vi "Configure Band Marker.vi"(0 "VISA resource name":refnum<visa-resource-name>, 1 "Enable Coupling (Disable)":bool, 2 "Sweep Type (1: Span/Center)":enum16{"Start/Stop", "Span/Center"}(ring)=enum."Span/Center", 3 "Start/Center (0)":dbl format="%^#_9g", 5 "Measurement Type (6: Phase Noise)":u16(ring)=6 items=["AM Noise"=1, "Baseband Noise"=2, "Freq/Power"=3, "Spectrum"=4, "Transient"=5, "Phase Noise"=6, "User"=7], 7 "Select Trace (1: 1)":u16(ring)=1 items=["1"=1, "2"=2, "3"=3, "4"=4, "5"=5, "6"=6, "7"=7, "8"=8], 9 "Select Band Marker (0: Band Marker X)":enum16{"Band Marker X", "Band Marker Y"}(ring), 11 "error in (no error)":errorcluster, 12 "Enable Band Marker (Enable)":bool=TRUE, 13 "Stop/Span (2E12)":dbl=2000000000000.0 format="%^#_9g") -> (4 "VISA resource name out":refnum<visa-resource-name>, 15 "error out":errorcluster)   [LabVIEW 2011, in "Agilent E5052X.lvlib"]
doc: "Configures band markers to be used in measurements. Band markers can be used to limit the range in which analysis or limit test measurements are taken."
uses:
  Agilent E5052X.lvlib
panel:
  # "Band Marker Settings"
  # "Band Marker Sweep Settings"
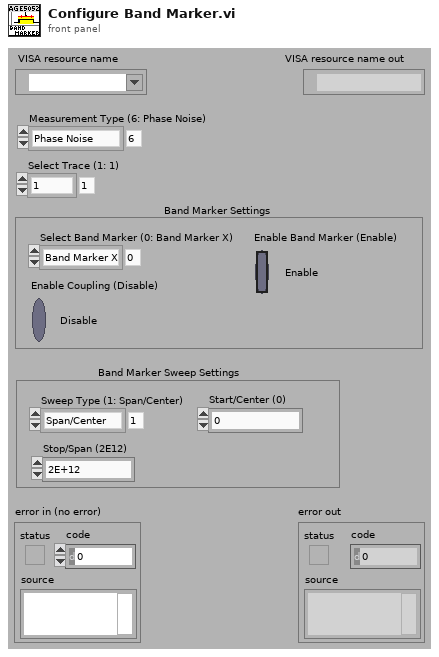
[diagram p1: front panel]
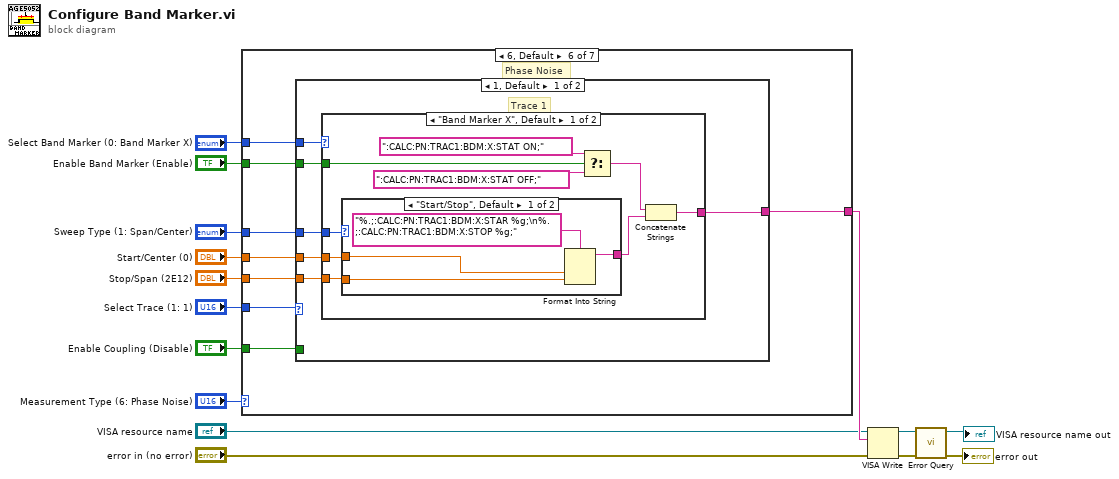
[diagram p0: block diagram]
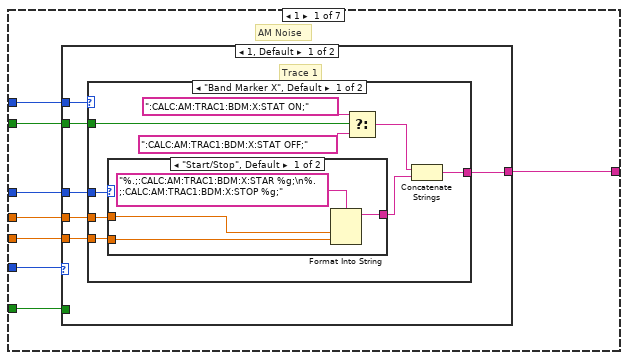
[diagram p2: hidden frame]
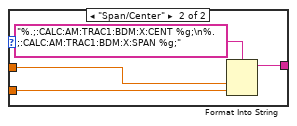
[diagram p3: hidden frame]
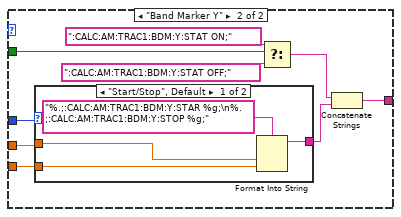
[diagram p4: hidden frame]
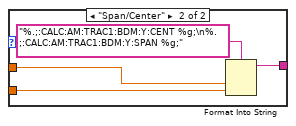
[diagram p5: hidden frame]
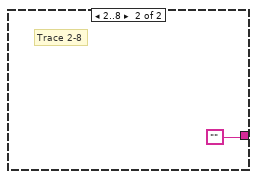
[diagram p6: hidden frame]
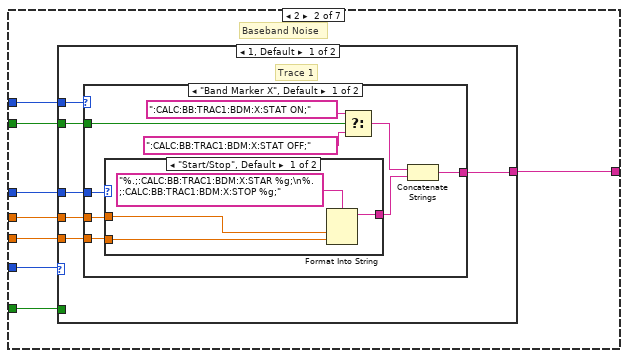
[diagram p7: hidden frame]
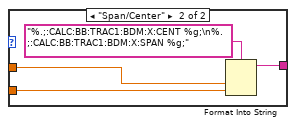
[diagram p8: hidden frame]
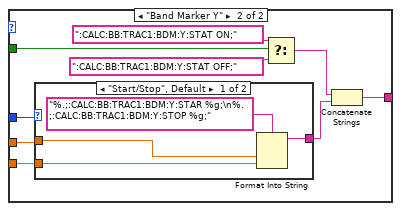
[diagram p9: hidden frame]
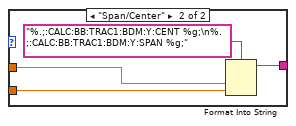
[diagram p10: hidden frame]
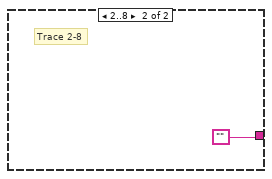
[diagram p11: hidden frame]
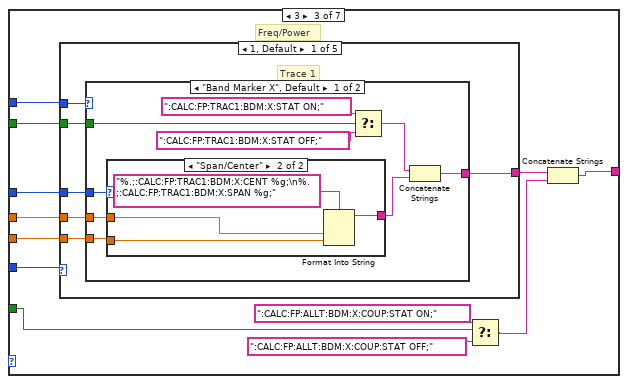
[diagram p12: hidden frame]
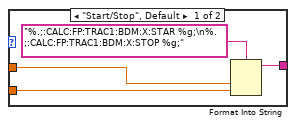
[diagram p13: hidden frame]
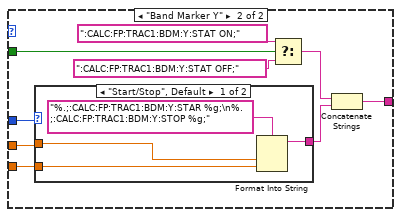
[diagram p14: hidden frame]
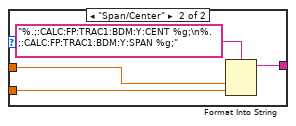
[diagram p15: hidden frame]
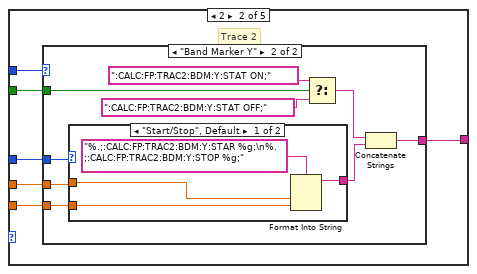
[diagram p16: hidden frame]
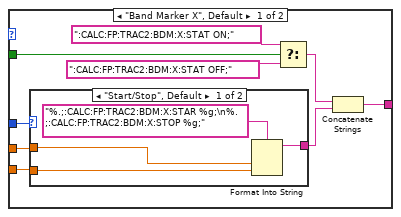
[diagram p17: hidden frame]
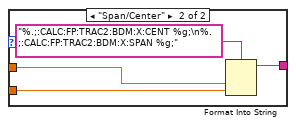
[diagram p18: hidden frame]
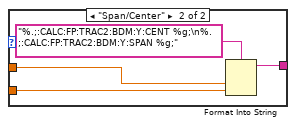
[diagram p19: hidden frame]
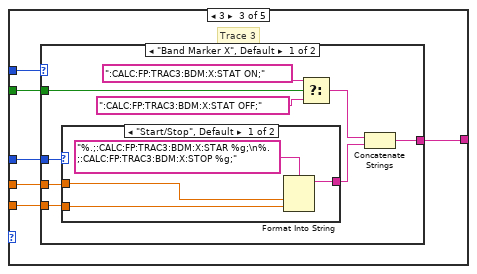
[diagram p20: hidden frame]
diagram:
  n1 = case shown="6, Default" "Measurement Type (6: Phase Noise)" {
    tunnel: "Select Band Marker (0: Band Marker X)" -> [w23 w72 w125 w289 w347 w516 w568]
    tunnel: "Select Trace (1: 1)" -> [w22 w67 w121 w293 w343 w512 w565]
    tunnel: "Enable Coupling (Disable)" -> [w21 w68 w115 w294 w337 w511 w559]
    tunnel: "Start/Center (0)" -> [w20 w70 w123 w291 w345 w514 w566]
    tunnel: "Stop/Span (2E12)" -> [w19 w69 w122 w292 w344 w513 w564]
    tunnel: "Sweep Type (1: Span/Center)" -> [w18 w71 w124 w290 w346 w515 w567]
    tunnel: [w17 w66 w120 w288 w342 w510 w569] -> w7
    tunnel: "Enable Band Marker (Enable)" -> [w16 w65 w118 w287 w340 w509 w562]
    frame 1 {
      # "AM Noise"
      n2 = case shown="1, Default" w22 {
        tunnel: w23 -> [w29 _]
        tunnel: w21 -> [_ _]
        tunnel: w20 -> [w27 _]
        tunnel: w19 -> [w26 _]
        tunnel: w18 -> [w28 _]
        tunnel: [w25 ""] -> w17
        tunnel: w16 -> [w24 _]
        frame 1, Default {
          # "Trace 1"
          n3 = case shown="\"Band Marker X\", Default" w29 {
            tunnel: w28 -> [w38 w55]
            tunnel: w27 -> [w37 w54]
            tunnel: w26 -> [w36 w53]
            tunnel: [w35 w51] -> w25
            tunnel: w24 -> [w32 w48]
            frame "Band Marker X", Default {
              n4 = case shown="\"Start/Stop\", Default" w38 {
                tunnel: w37 -> [w41 w45]
                tunnel: w36 -> [w42 w44]
                tunnel: [w39 w43] -> w34
                frame "Start/Stop", Default {
                  n5 = Format Into String(format string="%.;:CALC:AM:TRAC1:BDM:X:STAR %g;\n%.;:CALC:AM:TRAC1:BDM:X:STOP %g;", w41, w42) -> (resulting string=w39:string)  [unwired: 2 in, 1 out]
                }
                frame "Span/Center" {
                  n6 = Format Into String(format string="%.;:CALC:AM:TRAC1:BDM:X:CENT %g;\n%.;:CALC:AM:TRAC1:BDM:X:SPAN %g;", w45, w44) -> (resulting string=w43:string)  [unwired: 2 in, 1 out]
                }
              }
              n7 = Select(t=":CALC:AM:TRAC1:BDM:X:STAT ON;", s=w32, f=":CALC:AM:TRAC1:BDM:X:STAT OFF;") -> (s? t:f=w31:string)
              n8 = Concatenate Strings(w31, w34) -> (w35:string)
            }
            frame "Band Marker Y" {
              n9 = case shown="\"Start/Stop\", Default" w55 {
                tunnel: w54 -> [w58 w62]
                tunnel: w53 -> [w59 w61]
                tunnel: [w56 w60] -> w52
                frame "Start/Stop", Default {
                  n10 = Format Into String(format string="%.;:CALC:AM:TRAC1:BDM:Y:STAR %g;\n%.;:CALC:AM:TRAC1:BDM:Y:STOP %g;", w58, w59) -> (resulting string=w56:string)  [unwired: 2 in, 1 out]
                }
                frame "Span/Center" {
                  n11 = Format Into String(format string="%.;:CALC:AM:TRAC1:BDM:Y:CENT %g;\n%.;:CALC:AM:TRAC1:BDM:Y:SPAN %g;", w62, w61) -> (resulting string=w60:string)  [unwired: 2 in, 1 out]
                }
              }
              n12 = Select(t=":CALC:AM:TRAC1:BDM:Y:STAT ON;", s=w48, f=":CALC:AM:TRAC1:BDM:Y:STAT OFF;") -> (s? t:f=w47:string)
              n13 = Concatenate Strings(w47, w52) -> (w51:string)
            }
          }
        }
        frame 2..8 {
          # "Trace 2-8"
        }
      }
    }
    frame 2 {
      # "Baseband Noise"
      n14 = case shown="1, Default" w67 {
        tunnel: w72 -> [w78 _]
        tunnel: w68 -> [_ _]
        tunnel: w70 -> [w76 _]
        tunnel: w69 -> [w75 _]
        tunnel: w71 -> [w77 _]
        tunnel: [w74 ""] -> w66
        tunnel: w65 -> [w73 _]
        frame 1, Default {
          # "Trace 1"
          n15 = case shown="\"Band Marker X\", Default" w78 {
            tunnel: w77 -> [w87 w104]
            tunnel: w76 -> [w86 w103]
            tunnel: w75 -> [w85 w102]
            tunnel: [w84 w100] -> w74
            tunnel: w73 -> [w80 w97]
            frame "Band Marker X", Default {
              n16 = case shown="\"Start/Stop\", Default" w87 {
                tunnel: w86 -> [w90 w94]
                tunnel: w85 -> [w91 w93]
                tunnel: [w88 w92] -> w83
                frame "Start/Stop", Default {
                  n17 = Format Into String(format string="%.;:CALC:BB:TRAC1:BDM:X:STAR %g;\n%.;:CALC:BB:TRAC1:BDM:X:STOP %g;", w90, w91) -> (resulting string=w88:string)  [unwired: 2 in, 1 out]
                }
                frame "Span/Center" {
                  n18 = Format Into String(format string="%.;:CALC:BB:TRAC1:BDM:X:CENT %g;\n%.;:CALC:BB:TRAC1:BDM:X:SPAN %g;", w94, w93) -> (resulting string=w92:string)  [unwired: 2 in, 1 out]
                }
              }
              n19 = Select(t=":CALC:BB:TRAC1:BDM:X:STAT ON;", s=w80, f=":CALC:BB:TRAC1:BDM:X:STAT OFF;") -> (s? t:f=w79:string)
              n20 = Concatenate Strings(w79, w83) -> (w84:string)
            }
            frame "Band Marker Y" {
              n21 = case shown="\"Start/Stop\", Default" w104 {
                tunnel: w103 -> [w107 w111]
                tunnel: w102 -> [w108 w110]
                tunnel: [w105 w109] -> w101
                frame "Start/Stop", Default {
                  n22 = Format Into String(format string="%.;:CALC:BB:TRAC1:BDM:Y:STAR %g;\n%.;:CALC:BB:TRAC1:BDM:Y:STOP %g;", w107, w108) -> (resulting string=w105:string)  [unwired: 2 in, 1 out]
                }
                frame "Span/Center" {
                  n23 = Format Into String(format string="%.;:CALC:BB:TRAC1:BDM:Y:CENT %g;\n%.;:CALC:BB:TRAC1:BDM:Y:SPAN %g;", w111, w110) -> (resulting string=w109:string)  [unwired: 2 in, 1 out]
                }
              }
              n24 = Select(t=":CALC:BB:TRAC1:BDM:Y:STAT ON;", s=w97, f=":CALC:BB:TRAC1:BDM:Y:STAT OFF;") -> (s? t:f=w96:string)
              n25 = Concatenate Strings(w96, w101) -> (w100:string)
            }
          }
        }
        frame 2..8 {
          # "Trace 2-8"
        }
      }
    }
    frame 3 {
      # "Freq/Power"
      n26 = case shown="1, Default" w121 {
        tunnel: w125 -> [w131 w171 w210 w251 _]
        tunnel: w123 -> [w129 w169 w208 w249 _]
        tunnel: w122 -> [w128 w168 w207 w248 _]
        tunnel: w124 -> [w130 w170 w209 w250 _]
        tunnel: [w127 w167 w211 w247 ""] -> w119
        tunnel: w118 -> [w126 w166 w206 w246 _]
        frame 1, Default {
          # "Trace 1"
          n27 = case shown="\"Band Marker X\", Default" w131 {
            tunnel: w130 -> [w140 w157]
            tunnel: w129 -> [w139 w156]
            tunnel: w128 -> [w138 w155]
            tunnel: [w137 w153] -> w127
            tunnel: w126 -> [w133 w150]
            frame "Band Marker X", Default {
              n28 = case shown="\"Span/Center\"" w140 {
                tunnel: w139 -> [w143 w147]
                tunnel: w138 -> [w144 w146]
                tunnel: [w141 w145] -> w136
                frame "Start/Stop", Default {
                  n29 = Format Into String(format string="%.;:CALC:FP:TRAC1:BDM:X:STAR %g;\n%.;:CALC:FP:TRAC1:BDM:X:STOP %g;", w143, w144) -> (resulting string=w141:string)  [unwired: 2 in, 1 out]
                }
                frame "Span/Center" {
                  n30 = Format Into String(format string="%.;:CALC:FP:TRAC1:BDM:X:CENT %g;\n%.;:CALC:FP:TRAC1:BDM:X:SPAN %g;", w147, w146) -> (resulting string=w145:string)  [unwired: 2 in, 1 out]
                }
              }
              n31 = Select(t=":CALC:FP:TRAC1:BDM:X:STAT ON;", s=w133, f=":CALC:FP:TRAC1:BDM:X:STAT OFF;") -> (s? t:f=w132:string)
              n32 = Concatenate Strings(w132, w136) -> (w137:string)
            }
            frame "Band Marker Y" {
              n33 = case shown="\"Start/Stop\", Default" w157 {
                tunnel: w156 -> [w160 w164]
                tunnel: w155 -> [w161 w163]
                tunnel: [w158 w162] -> w154
                frame "Start/Stop", Default {
                  n34 = Format Into String(format string="%.;:CALC:FP:TRAC1:BDM:Y:STAR %g;\n%.;:CALC:FP:TRAC1:BDM:Y:STOP %g;", w160, w161) -> (resulting string=w158:string)  [unwired: 2 in, 1 out]
                }
                frame "Span/Center" {
                  n35 = Format Into String(format string="%.;:CALC:FP:TRAC1:BDM:Y:CENT %g;\n%.;:CALC:FP:TRAC1:BDM:Y:SPAN %g;", w164, w163) -> (resulting string=w162:string)  [unwired: 2 in, 1 out]
                }
              }
              n36 = Select(t=":CALC:FP:TRAC1:BDM:Y:STAT ON;", s=w150, f=":CALC:FP:TRAC1:BDM:Y:STAT OFF;") -> (s? t:f=w149:string)
              n37 = Concatenate Strings(w149, w154) -> (w153:string)
            }
          }
        }
        frame 2 {
          # "Trace 2"
          n38 = case shown="\"Band Marker Y\"" w171 {
            tunnel: w170 -> [w180 w197]
            tunnel: w169 -> [w179 w196]
            tunnel: w168 -> [w178 w195]
            tunnel: [w177 w193] -> w167
            tunnel: w166 -> [w173 w191]
            frame "Band Marker X", Default {
              n39 = case shown="\"Start/Stop\", Default" w180 {
                tunnel: w179 -> [w183 w187]
                tunnel: w178 -> [w184 w186]
                tunnel: [w181 w185] -> w176
                frame "Start/Stop", Default {
                  n40 = Format Into String(format string="%.;:CALC:FP:TRAC2:BDM:X:STAR %g;\n%.;:CALC:FP:TRAC2:BDM:X:STOP %g;", w183, w184) -> (resulting string=w181:string)  [unwired: 2 in, 1 out]
                }
                frame "Span/Center" {
                  n41 = Format Into String(format string="%.;:CALC:FP:TRAC2:BDM:X:CENT %g;\n%.;:CALC:FP:TRAC2:BDM:X:SPAN %g;", w187, w186) -> (resulting string=w185:string)  [unwired: 2 in, 1 out]
                }
              }
              n42 = Select(t=":CALC:FP:TRAC2:BDM:X:STAT ON;", s=w173, f=":CALC:FP:TRAC2:BDM:X:STAT OFF;") -> (s? t:f=w172:string)
              n43 = Concatenate Strings(w172, w176) -> (w177:string)
            }
            frame "Band Marker Y" {
              n44 = case shown="\"Start/Stop\", Default" w197 {
                tunnel: w196 -> [w200 w204]
                tunnel: w195 -> [w201 w203]
                tunnel: [w198 w202] -> w194
                frame "Start/Stop", Default {
                  n45 = Format Into String(format string="%.;:CALC:FP:TRAC2:BDM:Y:STAR %g;\n%.;:CALC:FP:TRAC2:BDM:Y:STOP %g;", w200, w201) -> (resulting string=w198:string)  [unwired: 2 in, 1 out]
                }
                frame "Span/Center" {
                  n46 = Format Into String(format string="%.;:CALC:FP:TRAC2:BDM:Y:CENT %g;\n%.;:CALC:FP:TRAC2:BDM:Y:SPAN %g;", w204, w203) -> (resulting string=w202:string)  [unwired: 2 in, 1 out]
                }
              }
              n47 = Select(t=":CALC:FP:TRAC2:BDM:Y:STAT ON;", s=w191, f=":CALC:FP:TRAC2:BDM:Y:STAT OFF;") -> (s? t:f=w190:string)
              n48 = Concatenate Strings(w190, w194) -> (w193:string)
            }
          }
        }
        frame 3 {
          # "Trace 3"
          n49 = case shown="\"Band Marker X\", Default" w210 {
            tunnel: w209 -> [w220 w237]
            tunnel: w208 -> [w219 w236]
            tunnel: w207 -> [w218 w235]
            tunnel: [w217 w233] -> w211
            tunnel: w206 -> [w213 w230]
            frame "Band Marker X", Default {
              n50 = case shown="\"Start/Stop\", Default" w220 {
                tunnel: w219 -> [w223 w227]
                tunnel: w218 -> [w224 w226]
                tunnel: [w221 w225] -> w216
                frame "Start/Stop", Default {
                  n51 = Format Into String(format string="%.;:CALC:FP:TRAC3:BDM:X:STAR %g;\n%.;:CALC:FP:TRAC3:BDM:X:STOP %g;", w223, w224) -> (resulting string=w221:string)  [unwired: 2 in, 1 out]
                }
                frame "Span/Center" {
                  n52 = Format Into String(format string="%.;:CALC:FP:TRAC3:BDM:X:CENT %g;\n%.;:CALC:FP:TRAC3:BDM:X:SPAN %g;", w227, w226) -> (resulting string=w225:string)  [unwired: 2 in, 1 out]
                }
              }
              n53 = Select(t=":CALC:FP:TRAC3:BDM:X:STAT ON;", s=w213, f=":CALC:FP:TRAC3:BDM:X:STAT OFF;") -> (s? t:f=w212:string)
              n54 = Concatenate Strings(w212, w216) -> (w217:string)
            }
            frame "Band Marker Y" {
              n55 = case shown="\"Start/Stop\", Default" w237 {
                tunnel: w236 -> [w240 w244]
                tunnel: w235 -> [w241 w243]
                tunnel: [w238 w242] -> w234
                frame "Start/Stop", Default {
                  n56 = Format Into String(format string="%.;:CALC:FP:TRAC3:BDM:Y:STAR %g;\n%.;:CALC:FP:TRAC3:BDM:Y:STOP %g;", w240, w241) -> (resulting string=w238:string)  [unwired: 2 in, 1 out]
                }
                frame "Span/Center" {
                  n57 = Format Into String(format string="%.;:CALC:FP:TRAC3:BDM:Y:CENT %g;\n%.;:CALC:FP:TRAC3:BDM:Y:SPAN %g;", w244, w243) -> (resulting string=w242:string)  [unwired: 2 in, 1 out]
                }
              }
              n58 = Select(t=":CALC:FP:TRAC3:BDM:Y:STAT ON;", s=w230, f=":CALC:FP:TRAC3:BDM:Y:STAT OFF;") -> (s? t:f=w229:string)
              n59 = Concatenate Strings(w229, w234) -> (w233:string)
            }
          }
        }
        frame 4 {
          # "Trace 4"
          n60 = case shown="\"Band Marker X\", Default" w251 {
            tunnel: w250 -> [w260 w277]
            tunnel: w249 -> [w259 w276]
            tunnel: w248 -> [w258 w275]
            tunnel: [w257 w273] -> w247
            tunnel: w246 -> [w253 w270]
            frame "Band Marker X", Default {
              n61 = case shown="\"Start/Stop\", Default" w260 {
                tunnel: w259 -> [w263 w267]
                tunnel: w258 -> [w264 w266]
                tunnel: [w261 w265] -> w256
                frame "Start/Stop", Default {
                  n62 = Format Into String(format string="%.;:CALC:FP:TRAC4:BDM:X:STAR %g;\n%.;:CALC:FP:TRAC4:BDM:X:STOP %g;", w263, w264) -> (resulting string=w261:string)  [unwired: 2 in, 1 out]
                }
                frame "Span/Center" {
                  n63 = Format Into String(format string="%.;:CALC:FP:TRAC4:BDM:X:CENT %g;\n%.;:CALC:FP:TRAC4:BDM:X:SPAN %g;", w267, w266) -> (resulting string=w265:string)  [unwired: 2 in, 1 out]
                }
              }
              n64 = Select(t=":CALC:FP:TRAC4:BDM:X:STAT ON;", s=w253, f=":CALC:FP:TRAC4:BDM:X:STAT OFF;") -> (s? t:f=w252:string)
              n65 = Concatenate Strings(w252, w256) -> (w257:string)
            }
            frame "Band Marker Y" {
              n66 = case shown="\"Start/Stop\", Default" w277 {
                tunnel: w276 -> [w280 w284]
                tunnel: w275 -> [w281 w283]
                tunnel: [w278 w282] -> w274
                frame "Start/Stop", Default {
                  n67 = Format Into String(format string="%.;:CALC:FP:TRAC4:BDM:Y:STAR %g;\n%.;:CALC:FP:TRAC4:BDM:Y:STOP %g;", w280, w281) -> (resulting string=w278:string)  [unwired: 2 in, 1 out]
                }
                frame "Span/Center" {
                  n68 = Format Into String(format string="%.;:CALC:FP:TRAC4:BDM:Y:CENT %g;\n%.;:CALC:FP:TRAC4:BDM:Y:SPAN %g;", w284, w283) -> (resulting string=w282:string)  [unwired: 2 in, 1 out]
                }
              }
              n69 = Select(t=":CALC:FP:TRAC4:BDM:Y:STAT ON;", s=w270, f=":CALC:FP:TRAC4:BDM:Y:STAT OFF;") -> (s? t:f=w269:string)
              n70 = Concatenate Strings(w269, w274) -> (w273:string)
            }
          }
        }
        frame 5..8 {
          # "Trace 5-8"
        }
      }
      n71 = Select(t=":CALC:FP:ALLT:BDM:X:COUP:STAT ON;", s=w115, f=":CALC:FP:ALLT:BDM:X:COUP:STAT OFF;") -> (s? t:f=w114:string)
      n72 = Concatenate Strings(w119, w114) -> (w120:string)
    }
    frame 4 {
      # "Spectrum Monitor"
      n73 = case shown="1, Default" w293 {
        tunnel: w289 -> [w300 _]
        tunnel: w294 -> [_ _]
        tunnel: w291 -> [w298 _]
        tunnel: w292 -> [w297 _]
        tunnel: w290 -> [w299 _]
        tunnel: [w296 ""] -> w288
        tunnel: w287 -> [w295 _]
        frame 1, Default {
          # "Trace 1"
          n74 = case shown="\"Band Marker X\", Default" w300 {
            tunnel: w299 -> [w309 w326]
            tunnel: w298 -> [w308 w325]
            tunnel: w297 -> [w307 w324]
            tunnel: [w306 w322] -> w296
            tunnel: w295 -> [w302 w320]
            frame "Band Marker X", Default {
              n75 = case shown="\"Span/Center\"" w309 {
                tunnel: w308 -> [w312 w316]
                tunnel: w307 -> [w313 w315]
                tunnel: [w310 w314] -> w305
                frame "Start/Stop", Default {
                  n76 = Format Into String(format string="%.;:CALC:SP:TRAC1:BDM:X:STAR %g;\n%.;:CALC:SP:TRAC1:BDM:X:STOP %g;", w312, w313) -> (resulting string=w310:string)  [unwired: 2 in, 1 out]
                }
                frame "Span/Center" {
                  n77 = Format Into String(format string="%.;:CALC:SP:TRAC1:BDM:X:CENT %g;\n%.;:CALC:SP:TRAC1:BDM:X:SPAN %g;", w316, w315) -> (resulting string=w314:string)  [unwired: 2 in, 1 out]
                }
              }
              n78 = Select(t=":CALC:SP:TRAC1:BDM:X:STAT ON;", s=w302, f=":CALC:SP:TRAC1:BDM:X:STAT OFF;") -> (s? t:f=w301:string)
              n79 = Concatenate Strings(w301, w305) -> (w306:string)
            }
            frame "Band Marker Y" {
              n80 = case shown="\"Start/Stop\", Default" w326 {
                tunnel: w325 -> [w329 w333]
                tunnel: w324 -> [w330 w332]
                tunnel: [w327 w331] -> w323
                frame "Start/Stop", Default {
                  n81 = Format Into String(format string="%.;:CALC:SP:TRAC1:BDM:Y:STAR %g;\n%.;:CALC:SP:TRAC1:BDM:Y:STOP %g;", w329, w330) -> (resulting string=w327:string)  [unwired: 2 in, 1 out]
                }
                frame "Span/Center" {
                  n82 = Format Into String(format string="%.;:CALC:SP:TRAC1:BDM:Y:CENT %g;\n%.;:CALC:SP:TRAC1:BDM:Y:SPAN %g;", w333, w332) -> (resulting string=w331:string)  [unwired: 2 in, 1 out]
                }
              }
              n83 = Select(t=":CALC:SP:TRAC1:BDM:Y:STAT ON;", s=w320, f=":CALC:SP:TRAC1:BDM:Y:STAT OFF;") -> (s? t:f=w319:string)
              n84 = Concatenate Strings(w319, w323) -> (w322:string)
            }
          }
        }
        frame 2..8 {
          # "Trace 2-8"
        }
      }
    }
    frame 5 {
      # "Transient"
      n85 = case shown="1, Default" w343 {
        tunnel: w347 -> [w353 w393 w432 w473 _]
        tunnel: w345 -> [w351 w391 w430 w471 _]
        tunnel: w344 -> [w350 w390 w429 w470 _]
        tunnel: w346 -> [w352 w392 w431 w472 _]
        tunnel: [w349 w389 w433 w469 ""] -> w341
        tunnel: w340 -> [w348 w388 w428 w468 _]
        frame 1, Default {
          # "Trace 1"
          n86 = case shown="\"Band Marker Y\"" w353 {
            tunnel: w352 -> [w362 w379]
            tunnel: w351 -> [w361 w378]
            tunnel: w350 -> [w360 w377]
            tunnel: [w359 w375] -> w349
            tunnel: w348 -> [w355 w372]
            frame "Band Marker X", Default {
              n87 = case shown="\"Start/Stop\", Default" w362 {
                tunnel: w361 -> [w365 w369]
                tunnel: w360 -> [w366 w368]
                tunnel: [w363 w367] -> w358
                frame "Start/Stop", Default {
                  n88 = Format Into String(format string="%.;:CALC:TR:TRAC1:BDM:X:STAR %g;\n%.;:CALC:TR:TRAC1:BDM:X:STOP %g;", w365, w366) -> (resulting string=w363:string)  [unwired: 2 in, 1 out]
                }
                frame "Span/Center" {
                  n89 = Format Into String(format string="%.;:CALC:TR:TRAC1:BDM:X:CENT %g;\n%.;:CALC:TR:TRAC1:BDM:X:SPAN %g;", w369, w368) -> (resulting string=w367:string)  [unwired: 2 in, 1 out]
                }
              }
              n90 = Select(t=":CALC:TR:TRAC1:BDM:X:STAT ON;", s=w355, f=":CALC:TR:TRAC1:BDM:X:STAT OFF;") -> (s? t:f=w354:string)
              n91 = Concatenate Strings(w354, w358) -> (w359:string)
            }
            frame "Band Marker Y" {
              n92 = case shown="\"Start/Stop\", Default" w379 {
                tunnel: w378 -> [w382 w386]
                tunnel: w377 -> [w383 w385]
                tunnel: [w380 w384] -> w376
                frame "Start/Stop", Default {
                  n93 = Format Into String(format string="%.;:CALC:TR:TRAC1:BDM:Y:STAR %g;\n%.;:CALC:TR:TRAC1:BDM:Y:STOP %g;", w382, w383) -> (resulting string=w380:string)  [unwired: 2 in, 1 out]
                }
                frame "Span/Center" {
                  n94 = Format Into String(format string="%.;:CALC:TR:TRAC1:BDM:Y:CENT %g;\n%.;:CALC:TR:TRAC1:BDM:Y:SPAN %g;", w386, w385) -> (resulting string=w384:string)  [unwired: 2 in, 1 out]
                }
              }
              n95 = Select(t=":CALC:TR:TRAC1:BDM:Y:STAT ON;", s=w372, f=":CALC:TR:TRAC1:BDM:Y:STAT OFF;") -> (s? t:f=w371:string)
              n96 = Concatenate Strings(w371, w376) -> (w375:string)
            }
          }
        }
        frame 2 {
          # "Trace 2"
          n97 = case shown="\"Band Marker Y\"" w393 {
            tunnel: w392 -> [w402 w419]
            tunnel: w391 -> [w401 w418]
            tunnel: w390 -> [w400 w417]
            tunnel: [w399 w415] -> w389
            tunnel: w388 -> [w395 w412]
            frame "Band Marker X", Default {
              n98 = case shown="\"Start/Stop\", Default" w402 {
                tunnel: w401 -> [w405 w409]
                tunnel: w400 -> [w406 w408]
                tunnel: [w403 w407] -> w398
                frame "Start/Stop", Default {
                  n99 = Format Into String(format string="%.;:CALC:TR:TRAC2:BDM:X:STAR %g;\n%.;:CALC:TR:TRAC2:BDM:X:STOP %g;", w405, w406) -> (resulting string=w403:string)  [unwired: 2 in, 1 out]
                }
                frame "Span/Center" {
                  n100 = Format Into String(format string="%.;:CALC:TR:TRAC2:BDM:X:CENT %g;\n%.;:CALC:TR:TRAC2:BDM:X:SPAN %g;", w409, w408) -> (resulting string=w407:string)  [unwired: 2 in, 1 out]
                }
              }
              n101 = Select(t=":CALC:TR:TRAC2:BDM:X:STAT ON;", s=w395, f=":CALC:TR:TRAC2:BDM:X:STAT OFF;") -> (s? t:f=w394:string)
              n102 = Concatenate Strings(w394, w398) -> (w399:string)
            }
            frame "Band Marker Y" {
              n103 = case shown="\"Start/Stop\", Default" w419 {
                tunnel: w418 -> [w422 w426]
                tunnel: w417 -> [w423 w425]
                tunnel: [w420 w424] -> w416
                frame "Start/Stop", Default {
                  n104 = Format Into String(format string="%.;:CALC:TR:TRAC2:BDM:Y:STAR %g;\n%.;:CALC:TR:TRAC2:BDM:Y:STOP %g;", w422, w423) -> (resulting string=w420:string)  [unwired: 2 in, 1 out]
                }
                frame "Span/Center" {
                  n105 = Format Into String(format string="%.;:CALC:TR:TRAC2:BDM:Y:CENT %g;\n%.;:CALC:TR:TRAC2:BDM:Y:SPAN %g;", w426, w425) -> (resulting string=w424:string)  [unwired: 2 in, 1 out]
                }
              }
              n106 = Select(t=":CALC:TR:TRAC2:BDM:Y:STAT ON;", s=w412, f=":CALC:TR:TRAC2:BDM:Y:STAT OFF;") -> (s? t:f=w411:string)
              n107 = Concatenate Strings(w411, w416) -> (w415:string)
            }
          }
        }
        frame 3 {
          # "Trace 3"
          n108 = case shown="\"Band Marker X\", Default" w432 {
            tunnel: w431 -> [w442 w459]
            tunnel: w430 -> [w441 w458]
            tunnel: w429 -> [w440 w457]
            tunnel: [w439 w455] -> w433
            tunnel: w428 -> [w435 w452]
            frame "Band Marker X", Default {
              n109 = case shown="\"Start/Stop\", Default" w442 {
                tunnel: w441 -> [w445 w449]
                tunnel: w440 -> [w446 w448]
                tunnel: [w443 w447] -> w438
                frame "Start/Stop", Default {
                  n110 = Format Into String(format string="%.;:CALC:TR:TRAC3:BDM:X:STAR %g;\n%.;:CALC:TR:TRAC3:BDM:X:STOP %g;", w445, w446) -> (resulting string=w443:string)  [unwired: 2 in, 1 out]
                }
                frame "Span/Center" {
                  n111 = Format Into String(format string="%.;:CALC:TR:TRAC3:BDM:X:CENT %g;\n%.;:CALC:TR:TRAC3:BDM:X:SPAN %g;", w449, w448) -> (resulting string=w447:string)  [unwired: 2 in, 1 out]
                }
              }
              n112 = Select(t=":CALC:TR:TRAC3:BDM:X:STAT ON;", s=w435, f=":CALC:TR:TRAC3:BDM:X:STAT OFF;") -> (s? t:f=w434:string)
              n113 = Concatenate Strings(w434, w438) -> (w439:string)
            }
            frame "Band Marker Y" {
              n114 = case shown="\"Start/Stop\", Default" w459 {
                tunnel: w458 -> [w462 w466]
                tunnel: w457 -> [w463 w465]
                tunnel: [w460 w464] -> w456
                frame "Start/Stop", Default {
                  n115 = Format Into String(format string="%.;:CALC:TR:TRAC3:BDM:Y:STAR %g;\n%.;:CALC:TR:TRAC3:BDM:Y:STOP %g;", w462, w463) -> (resulting string=w460:string)  [unwired: 2 in, 1 out]
                }
                frame "Span/Center" {
                  n116 = Format Into String(format string="%.;:CALC:TR:TRAC3:BDM:Y:CENT %g;\n%.;:CALC:TR:TRAC3:BDM:Y:SPAN %g;", w466, w465) -> (resulting string=w464:string)  [unwired: 2 in, 1 out]
                }
              }
              n117 = Select(t=":CALC:TR:TRAC3:BDM:Y:STAT ON;", s=w452, f=":CALC:TR:TRAC3:BDM:Y:STAT OFF;") -> (s? t:f=w451:string)
              n118 = Concatenate Strings(w451, w456) -> (w455:string)
            }
          }
        }
        frame 4 {
          # "Trace 4"
          n119 = case shown="\"Band Marker X\", Default" w473 {
            tunnel: w472 -> [w482 w499]
            tunnel: w471 -> [w481 w498]
            tunnel: w470 -> [w480 w497]
            tunnel: [w479 w495] -> w469
            tunnel: w468 -> [w475 w492]
            frame "Band Marker X", Default {
              n120 = case shown="\"Start/Stop\", Default" w482 {
                tunnel: w481 -> [w485 w489]
                tunnel: w480 -> [w486 w488]
                tunnel: [w483 w487] -> w478
                frame "Start/Stop", Default {
                  n121 = Format Into String(format string="%.;:CALC:TR:TRAC4:BDM:X:STAR %g;\n%.;:CALC:TR:TRAC4:BDM:X:STOP %g;", w485, w486) -> (resulting string=w483:string)  [unwired: 2 in, 1 out]
                }
                frame "Span/Center" {
                  n122 = Format Into String(format string="%.;:CALC:TR:TRAC4:BDM:X:CENT %g;\n%.;:CALC:TR:TRAC4:BDM:X:SPAN %g;", w489, w488) -> (resulting string=w487:string)  [unwired: 2 in, 1 out]
                }
              }
              n123 = Select(t=":CALC:TR:TRAC4:BDM:X:STAT ON;", s=w475, f=":CALC:TR:TRAC4:BDM:X:STAT OFF;") -> (s? t:f=w474:string)
              n124 = Concatenate Strings(w474, w478) -> (w479:string)
            }
            frame "Band Marker Y" {
              n125 = case shown="\"Start/Stop\", Default" w499 {
                tunnel: w498 -> [w502 w506]
                tunnel: w497 -> [w503 w505]
                tunnel: [w500 w504] -> w496
                frame "Start/Stop", Default {
                  n126 = Format Into String(format string="%.;:CALC:TR:TRAC4:BDM:Y:STAR %g;\n%.;:CALC:TR:TRAC4:BDM:Y:STOP %g;", w502, w503) -> (resulting string=w500:string)  [unwired: 2 in, 1 out]
                }
                frame "Span/Center" {
                  n127 = Format Into String(format string="%.;:CALC:TR:TRAC4:BDM:Y:CENT %g;\n%.;:CALC:TR:TRAC4:BDM:Y:SPAN %g;", w506, w505) -> (resulting string=w504:string)  [unwired: 2 in, 1 out]
                }
              }
              n128 = Select(t=":CALC:TR:TRAC4:BDM:Y:STAT ON;", s=w492, f=":CALC:TR:TRAC4:BDM:Y:STAT OFF;") -> (s? t:f=w491:string)
              n129 = Concatenate Strings(w491, w496) -> (w495:string)
            }
          }
        }
        frame 5..8 {
          # "Trace 5-8"
        }
      }
      n130 = Select(t=":CALC:TR:ALLT:BDM:X:COUP:STAT ON;", s=w337, f=":CALC:TR:ALLT:BDM:X:COUP:STAT OFF;") -> (s? t:f=w336:string)
      n131 = Concatenate Strings(w341, w336) -> (w342:string)
    }
    frame 6, Default {
      # "Phase Noise"
      n132 = case shown="1, Default" w512 {
        tunnel: w516 -> [w522 _]
        tunnel: w511 -> [_ _]
        tunnel: w514 -> [w520 _]
        tunnel: w513 -> [w519 _]
        tunnel: w515 -> [w521 _]
        tunnel: [w518 ""] -> w510
        tunnel: w509 -> [w517 _]
        frame 1, Default {
          # "Trace 1"
          n133 = case shown="\"Band Marker X\", Default" w522 {
            tunnel: w521 -> [w531 w548]
            tunnel: w520 -> [w530 w547]
            tunnel: w519 -> [w529 w546]
            tunnel: [w528 w544] -> w518
            tunnel: w517 -> [w524 w541]
            frame "Band Marker X", Default {
              n134 = case shown="\"Start/Stop\", Default" w531 {
                tunnel: w530 -> [w534 w538]
                tunnel: w529 -> [w535 w537]
                tunnel: [w532 w536] -> w527
                frame "Start/Stop", Default {
                  n135 = Format Into String(format string="%.;:CALC:PN:TRAC1:BDM:X:STAR %g;\n%.;:CALC:PN:TRAC1:BDM:X:STOP %g;", w534, w535) -> (resulting string=w532:string)  [unwired: 2 in, 1 out]
                }
                frame "Span/Center" {
                  n136 = Format Into String(format string="%.;:CALC:PN:TRAC1:BDM:X:CENT %g;\n%.;:CALC:PN:TRAC1:BDM:X:SPAN %g;", w538, w537) -> (resulting string=w536:string)  [unwired: 2 in, 1 out]
                }
              }
              n137 = Select(t=":CALC:PN:TRAC1:BDM:X:STAT ON;", s=w524, f=":CALC:PN:TRAC1:BDM:X:STAT OFF;") -> (s? t:f=w523:string)
              n138 = Concatenate Strings(w523, w527) -> (w528:string)
            }
            frame "Band Marker Y" {
              n139 = case shown="\"Start/Stop\", Default" w548 {
                tunnel: w547 -> [w551 w555]
                tunnel: w546 -> [w552 w554]
                tunnel: [w549 w553] -> w545
                frame "Start/Stop", Default {
                  n140 = Format Into String(format string="%.;:CALC:PN:TRAC1:BDM:Y:STAR %g;\n%.;:CALC:PN:TRAC1:BDM:Y:STOP %g;", w551, w552) -> (resulting string=w549:string)  [unwired: 2 in, 1 out]
                }
                frame "Span/Center" {
                  n141 = Format Into String(format string="%.;:CALC:PN:TRAC1:BDM:Y:CENT %g;\n%.;:CALC:PN:TRAC1:BDM:Y:SPAN %g;", w555, w554) -> (resulting string=w553:string)  [unwired: 2 in, 1 out]
                }
              }
              n142 = Select(t=":CALC:PN:TRAC1:BDM:Y:STAT ON;", s=w541, f=":CALC:PN:TRAC1:BDM:Y:STAT OFF;") -> (s? t:f=w540:string)
              n143 = Concatenate Strings(w540, w545) -> (w544:string)
            }
          }
        }
        frame 2..8 {
          # "Trace 2-8"
        }
      }
    }
    frame 7 {
      # "User"
      n144 = case shown="1, Default" w565 {
        tunnel: w568 -> [w575 w615 w654 w695 w735 w775 w814 w855]
        tunnel: w566 -> [w573 w613 w652 w693 w733 w773 w812 w853]
        tunnel: w564 -> [w572 w612 w651 w692 w732 w772 w811 w852]
        tunnel: w567 -> [w574 w614 w653 w694 w734 w774 w813 w854]
        tunnel: [w571 w611 w655 w691 w731 w771 w815 w851] -> w563
        tunnel: w562 -> [w570 w610 w650 w690 w730 w770 w810 w850]
        frame 1, Default {
          # "Trace 1"
          n145 = case shown="\"Band Marker X\", Default" w575 {
            tunnel: w574 -> [w584 w601]
            tunnel: w573 -> [w583 w600]
            tunnel: w572 -> [w582 w599]
            tunnel: [w581 w597] -> w571
            tunnel: w570 -> [w577 w594]
            frame "Band Marker X", Default {
              n146 = case shown="\"Start/Stop\", Default" w584 {
                tunnel: w583 -> [w587 w591]
                tunnel: w582 -> [w588 w590]
                tunnel: [w585 w589] -> w580
                frame "Start/Stop", Default {
                  n147 = Format Into String(format string="%.;:CALC:USER:TRAC1:BDM:X:STAR %g;\n%.;:CALC:USER:TRAC1:BDM:X:STOP %g;", w587, w588) -> (resulting string=w585:string)  [unwired: 2 in, 1 out]
                }
                frame "Span/Center" {
                  n148 = Format Into String(format string="%.;:CALC:USER:TRAC1:BDM:X:CENT %g;\n%.;:CALC:USER:TRAC1:BDM:X:SPAN %g;", w591, w590) -> (resulting string=w589:string)  [unwired: 2 in, 1 out]
                }
              }
              n149 = Select(t=":CALC:USER:TRAC1:BDM:X:STAT ON;", s=w577, f=":CALC:USER:TRAC1:BDM:X:STAT OFF;") -> (s? t:f=w576:string)
              n150 = Concatenate Strings(w576, w580) -> (w581:string)
            }
            frame "Band Marker Y" {
              n151 = case shown="\"Start/Stop\", Default" w601 {
                tunnel: w600 -> [w604 w608]
                tunnel: w599 -> [w605 w607]
                tunnel: [w602 w606] -> w598
                frame "Start/Stop", Default {
                  n152 = Format Into String(format string="%.;:CALC:USER:TRAC1:BDM:Y:STAR %g;\n%.;:CALC:USER:TRAC1:BDM:Y:STOP %g;", w604, w605) -> (resulting string=w602:string)  [unwired: 2 in, 1 out]
                }
                frame "Span/Center" {
                  n153 = Format Into String(format string="%.;:CALC:USER:TRAC1:BDM:Y:CENT %g;\n%.;:CALC:USER:TRAC1:BDM:Y:SPAN %g;", w608, w607) -> (resulting string=w606:string)  [unwired: 2 in, 1 out]
                }
              }
              n154 = Select(t=":CALC:USER:TRAC1:BDM:Y:STAT ON;", s=w594, f=":CALC:USER:TRAC1:BDM:Y:STAT OFF;") -> (s? t:f=w593:string)
              n155 = Concatenate Strings(w593, w598) -> (w597:string)
            }
          }
        }
        frame 2 {
          # "Trace 2"
          n156 = case shown="\"Band Marker X\", Default" w615 {
            tunnel: w614 -> [w624 w641]
            tunnel: w613 -> [w623 w640]
            tunnel: w612 -> [w622 w639]
            tunnel: [w621 w637] -> w611
            tunnel: w610 -> [w617 w634]
            frame "Band Marker X", Default {
              n157 = case shown="\"Start/Stop\", Default" w624 {
                tunnel: w623 -> [w627 w631]
                tunnel: w622 -> [w628 w630]
                tunnel: [w625 w629] -> w620
                frame "Start/Stop", Default {
                  n158 = Format Into String(format string="%.;:CALC:USER:TRAC2:BDM:X:STAR %g;\n%.;:CALC:USER:TRAC2:BDM:X:STOP %g;", w627, w628) -> (resulting string=w625:string)  [unwired: 2 in, 1 out]
                }
                frame "Span/Center" {
                  n159 = Format Into String(format string="%.;:CALC:USER:TRAC2:BDM:X:CENT %g;\n%.;:CALC:USER:TRAC2:BDM:X:SPAN %g;", w631, w630) -> (resulting string=w629:string)  [unwired: 2 in, 1 out]
                }
              }
              n160 = Select(t=":CALC:USER:TRAC2:BDM:X:STAT ON;", s=w617, f=":CALC:USER:TRAC2:BDM:X:STAT OFF;") -> (s? t:f=w616:string)
              n161 = Concatenate Strings(w616, w620) -> (w621:string)
            }
            frame "Band Marker Y" {
              n162 = case shown="\"Start/Stop\", Default" w641 {
                tunnel: w640 -> [w644 w648]
                tunnel: w639 -> [w645 w647]
                tunnel: [w642 w646] -> w638
                frame "Start/Stop", Default {
                  n163 = Format Into String(format string="%.;:CALC:USER:TRAC2:BDM:Y:STAR %g;\n%.;:CALC:USER:TRAC2:BDM:Y:STOP %g;", w644, w645) -> (resulting string=w642:string)  [unwired: 2 in, 1 out]
                }
                frame "Span/Center" {
                  n164 = Format Into String(format string="%.;:CALC:USER:TRAC2:BDM:Y:CENT %g;\n%.;:CALC:USER:TRAC2:BDM:Y:SPAN %g;", w648, w647) -> (resulting string=w646:string)  [unwired: 2 in, 1 out]
                }
              }
              n165 = Select(t=":CALC:USER:TRAC2:BDM:Y:STAT ON;", s=w634, f=":CALC:USER:TRAC2:BDM:Y:STAT OFF;") -> (s? t:f=w633:string)
              n166 = Concatenate Strings(w633, w638) -> (w637:string)
            }
          }
        }
        frame 3 {
          # "Trace 3"
          n167 = case shown="\"Band Marker X\", Default" w654 {
            tunnel: w653 -> [w664 w681]
            tunnel: w652 -> [w663 w680]
            tunnel: w651 -> [w662 w679]
            tunnel: [w661 w677] -> w655
            tunnel: w650 -> [w657 w674]
            frame "Band Marker X", Default {
              n168 = case shown="\"Start/Stop\", Default" w664 {
                tunnel: w663 -> [w667 w671]
                tunnel: w662 -> [w668 w670]
                tunnel: [w665 w669] -> w660
                frame "Start/Stop", Default {
                  n169 = Format Into String(format string="%.;:CALC:USER:TRAC3:BDM:X:STAR %g;\n%.;:CALC:USER:TRAC3:BDM:X:STOP %g;", w667, w668) -> (resulting string=w665:string)  [unwired: 2 in, 1 out]
                }
                frame "Span/Center" {
                  n170 = Format Into String(format string="%.;:CALC:USER:TRAC3:BDM:X:CENT %g;\n%.;:CALC:USER:TRAC3:BDM:X:SPAN %g;", w671, w670) -> (resulting string=w669:string)  [unwired: 2 in, 1 out]
                }
              }
              n171 = Select(t=":CALC:USER:TRAC3:BDM:X:STAT ON;", s=w657, f=":CALC:USER:TRAC3:BDM:X:STAT OFF;") -> (s? t:f=w656:string)
              n172 = Concatenate Strings(w656, w660) -> (w661:string)
            }
            frame "Band Marker Y" {
              n173 = case shown="\"Start/Stop\", Default" w681 {
                tunnel: w680 -> [w684 w688]
                tunnel: w679 -> [w685 w687]
                tunnel: [w682 w686] -> w678
                frame "Start/Stop", Default {
                  n174 = Format Into String(format string="%.;:CALC:USER:TRAC3:BDM:Y:STAR %g;\n%.;:CALC:USER:TRAC3:BDM:Y:STOP %g;", w684, w685) -> (resulting string=w682:string)  [unwired: 2 in, 1 out]
                }
                frame "Span/Center" {
                  n175 = Format Into String(format string="%.;:CALC:USER:TRAC3:BDM:Y:CENT %g;\n%.;:CALC:USER:TRAC3:BDM:Y:SPAN %g;", w688, w687) -> (resulting string=w686:string)  [unwired: 2 in, 1 out]
                }
              }
              n176 = Select(t=":CALC:USER:TRAC3:BDM:Y:STAT ON;", s=w674, f=":CALC:USER:TRAC3:BDM:Y:STAT OFF;") -> (s? t:f=w673:string)
              n177 = Concatenate Strings(w673, w678) -> (w677:string)
            }
          }
        }
        frame 4 {
          # "Trace 4"
          n178 = case shown="\"Band Marker X\", Default" w695 {
            tunnel: w694 -> [w704 w721]
            tunnel: w693 -> [w703 w720]
            tunnel: w692 -> [w702 w719]
            tunnel: [w701 w717] -> w691
            tunnel: w690 -> [w697 w714]
            frame "Band Marker X", Default {
              n179 = case shown="\"Start/Stop\", Default" w704 {
                tunnel: w703 -> [w707 w711]
                tunnel: w702 -> [w708 w710]
                tunnel: [w705 w709] -> w700
                frame "Start/Stop", Default {
                  n180 = Format Into String(format string="%.;:CALC:USER:TRAC4:BDM:X:STAR %g;\n%.;:CALC:USER:TRAC4:BDM:X:STOP %g;", w707, w708) -> (resulting string=w705:string)  [unwired: 2 in, 1 out]
                }
                frame "Span/Center" {
                  n181 = Format Into String(format string="%.;:CALC:USER:TRAC4:BDM:X:CENT %g;\n%.;:CALC:USER:TRAC4:BDM:X:SPAN %g;", w711, w710) -> (resulting string=w709:string)  [unwired: 2 in, 1 out]
                }
              }
              n182 = Select(t=":CALC:USER:TRAC4:BDM:X:STAT ON;", s=w697, f=":CALC:USER:TRAC4:BDM:X:STAT OFF;") -> (s? t:f=w696:string)
              n183 = Concatenate Strings(w696, w700) -> (w701:string)
            }
            frame "Band Marker Y" {
              n184 = case shown="\"Start/Stop\", Default" w721 {
                tunnel: w720 -> [w724 w728]
                tunnel: w719 -> [w725 w727]
                tunnel: [w722 w726] -> w718
                frame "Start/Stop", Default {
                  n185 = Format Into String(format string="%.;:CALC:USER:TRAC4:BDM:Y:STAR %g;\n%.;:CALC:USER:TRAC4:BDM:Y:STOP %g;", w724, w725) -> (resulting string=w722:string)  [unwired: 2 in, 1 out]
                }
                frame "Span/Center" {
                  n186 = Format Into String(format string="%.;:CALC:USER:TRAC4:BDM:Y:CENT %g;\n%.;:CALC:USER:TRAC4:BDM:Y:SPAN %g;", w728, w727) -> (resulting string=w726:string)  [unwired: 2 in, 1 out]
                }
              }
              n187 = Select(t=":CALC:USER:TRAC4:BDM:Y:STAT ON;", s=w714, f=":CALC:USER:TRAC4:BDM:Y:STAT OFF;") -> (s? t:f=w713:string)
              n188 = Concatenate Strings(w713, w718) -> (w717:string)
            }
          }
        }
        frame 5 {
          # "Trace 5"
          n189 = case shown="\"Band Marker X\", Default" w735 {
            tunnel: w734 -> [w744 w761]
            tunnel: w733 -> [w743 w760]
            tunnel: w732 -> [w742 w759]
            tunnel: [w741 w757] -> w731
            tunnel: w730 -> [w737 w754]
            frame "Band Marker X", Default {
              n190 = case shown="\"Start/Stop\", Default" w744 {
                tunnel: w743 -> [w747 w751]
                tunnel: w742 -> [w748 w750]
                tunnel: [w745 w749] -> w740
                frame "Start/Stop", Default {
                  n191 = Format Into String(format string="%.;:CALC:USER:TRAC5:BDM:X:STAR %g;\n%.;:CALC:USER:TRAC5:BDM:X:STOP %g;", w747, w748) -> (resulting string=w745:string)  [unwired: 2 in, 1 out]
                }
                frame "Span/Center" {
                  n192 = Format Into String(format string="%.;:CALC:USER:TRAC5:BDM:X:CENT %g;\n%.;:CALC:USER:TRAC5:BDM:X:SPAN %g;", w751, w750) -> (resulting string=w749:string)  [unwired: 2 in, 1 out]
                }
              }
              n193 = Select(t=":CALC:USER:TRAC5:BDM:X:STAT ON;", s=w737, f=":CALC:USER:TRAC5:BDM:X:STAT OFF;") -> (s? t:f=w736:string)
              n194 = Concatenate Strings(w736, w740) -> (w741:string)
            }
            frame "Band Marker Y" {
              n195 = case shown="\"Start/Stop\", Default" w761 {
                tunnel: w760 -> [w764 w768]
                tunnel: w759 -> [w765 w767]
                tunnel: [w762 w766] -> w758
                frame "Start/Stop", Default {
                  n196 = Format Into String(format string="%.;:CALC:USER:TRAC5:BDM:Y:STAR %g;\n%.;:CALC:USER:TRAC5:BDM:Y:STOP %g;", w764, w765) -> (resulting string=w762:string)  [unwired: 2 in, 1 out]
                }
                frame "Span/Center" {
                  n197 = Format Into String(format string="%.;:CALC:USER:TRAC5:BDM:Y:CENT %g;\n%.;:CALC:USER:TRAC5:BDM:Y:SPAN %g;", w768, w767) -> (resulting string=w766:string)  [unwired: 2 in, 1 out]
                }
              }
              n198 = Select(t=":CALC:USER:TRAC5:BDM:Y:STAT ON;", s=w754, f=":CALC:USER:TRAC5:BDM:Y:STAT OFF;") -> (s? t:f=w753:string)
              n199 = Concatenate Strings(w753, w758) -> (w757:string)
            }
          }
        }
        frame 6 {
          # "Trace 6"
          n200 = case shown="\"Band Marker X\", Default" w775 {
            tunnel: w774 -> [w784 w801]
            tunnel: w773 -> [w783 w800]
            tunnel: w772 -> [w782 w799]
            tunnel: [w781 w797] -> w771
            tunnel: w770 -> [w777 w794]
            frame "Band Marker X", Default {
              n201 = case shown="\"Start/Stop\", Default" w784 {
                tunnel: w783 -> [w787 w791]
                tunnel: w782 -> [w788 w790]
                tunnel: [w785 w789] -> w780
                frame "Start/Stop", Default {
                  n202 = Format Into String(format string="%.;:CALC:USER:TRAC6:BDM:X:STAR %g;\n%.;:CALC:USER:TRAC6:BDM:X:STOP %g;", w787, w788) -> (resulting string=w785:string)  [unwired: 2 in, 1 out]
                }
                frame "Span/Center" {
                  n203 = Format Into String(format string="%.;:CALC:USER:TRAC6:BDM:X:CENT %g;\n%.;:CALC:USER:TRAC6:BDM:X:SPAN %g;", w791, w790) -> (resulting string=w789:string)  [unwired: 2 in, 1 out]
                }
              }
              n204 = Select(t=":CALC:USER:TRAC6:BDM:X:STAT ON;", s=w777, f=":CALC:USER:TRAC6:BDM:X:STAT OFF;") -> (s? t:f=w776:string)
              n205 = Concatenate Strings(w776, w780) -> (w781:string)
            }
            frame "Band Marker Y" {
              n206 = case shown="\"Start/Stop\", Default" w801 {
                tunnel: w800 -> [w804 w808]
                tunnel: w799 -> [w805 w807]
                tunnel: [w802 w806] -> w798
                frame "Start/Stop", Default {
                  n207 = Format Into String(format string="%.;:CALC:USER:TRAC6:BDM:Y:STAR %g;\n%.;:CALC:USER:TRAC6:BDM:Y:STOP %g;", w804, w805) -> (resulting string=w802:string)  [unwired: 2 in, 1 out]
                }
                frame "Span/Center" {
                  n208 = Format Into String(format string="%.;:CALC:USER:TRAC6:BDM:Y:CENT %g;\n%.;:CALC:USER:TRAC6:BDM:Y:SPAN %g;", w808, w807) -> (resulting string=w806:string)  [unwired: 2 in, 1 out]
                }
              }
              n209 = Select(t=":CALC:USER:TRAC6:BDM:Y:STAT ON;", s=w794, f=":CALC:USER:TRAC6:BDM:Y:STAT OFF;") -> (s? t:f=w793:string)
              n210 = Concatenate Strings(w793, w798) -> (w797:string)
            }
          }
        }
        frame 7 {
          # "Trace 7"
          n211 = case shown="\"Band Marker Y\"" w814 {
            tunnel: w813 -> [w824 w841]
            tunnel: w812 -> [w823 w840]
            tunnel: w811 -> [w822 w839]
            tunnel: [w821 w837] -> w815
            tunnel: w810 -> [w817 w834]
            frame "Band Marker X", Default {
              n212 = case shown="\"Start/Stop\", Default" w824 {
                tunnel: w823 -> [w827 w831]
                tunnel: w822 -> [w828 w830]
                tunnel: [w825 w829] -> w820
                frame "Start/Stop", Default {
                  n213 = Format Into String(format string="%.;:CALC:USER:TRAC7:BDM:X:STAR %g;\n%.;:CALC:USER:TRAC7:BDM:X:STOP %g;", w827, w828) -> (resulting string=w825:string)  [unwired: 2 in, 1 out]
                }
                frame "Span/Center" {
                  n214 = Format Into String(format string="%.;:CALC:USER:TRAC7:BDM:X:CENT %g;\n%.;:CALC:USER:TRAC7:BDM:X:SPAN %g;", w831, w830) -> (resulting string=w829:string)  [unwired: 2 in, 1 out]
                }
              }
              n215 = Select(t=":CALC:USER:TRAC7:BDM:X:STAT ON;", s=w817, f=":CALC:USER:TRAC7:BDM:X:STAT OFF;") -> (s? t:f=w816:string)
              n216 = Concatenate Strings(w816, w820) -> (w821:string)
            }
            frame "Band Marker Y" {
              n217 = case shown="\"Start/Stop\", Default" w841 {
                tunnel: w840 -> [w844 w848]
                tunnel: w839 -> [w845 w847]
                tunnel: [w842 w846] -> w838
                frame "Start/Stop", Default {
                  n218 = Format Into String(format string="%.;:CALC:USER:TRAC7:BDM:Y:STAR %g;\n%.;:CALC:USER:TRAC7:BDM:Y:STOP %g;", w844, w845) -> (resulting string=w842:string)  [unwired: 2 in, 1 out]
                }
                frame "Span/Center" {
                  n219 = Format Into String(format string="%.;:CALC:USER:TRAC7:BDM:Y:CENT %g;\n%.;:CALC:USER:TRAC7:BDM:Y:SPAN %g;", w848, w847) -> (resulting string=w846:string)  [unwired: 2 in, 1 out]
                }
              }
              n220 = Select(t=":CALC:USER:TRAC7:BDM:Y:STAT ON;", s=w834, f=":CALC:USER:TRAC7:BDM:Y:STAT OFF;") -> (s? t:f=w833:string)
              n221 = Concatenate Strings(w833, w838) -> (w837:string)
            }
          }
        }
        frame 8 {
          # "Trace 8"
          n222 = case shown="\"Band Marker X\", Default" w855 {
            tunnel: w854 -> [w864 w881]
            tunnel: w853 -> [w863 w880]
            tunnel: w852 -> [w862 w879]
            tunnel: [w861 w877] -> w851
            tunnel: w850 -> [w857 w874]
            frame "Band Marker X", Default {
              n223 = case shown="\"Start/Stop\", Default" w864 {
                tunnel: w863 -> [w867 w871]
                tunnel: w862 -> [w868 w870]
                tunnel: [w865 w869] -> w860
                frame "Start/Stop", Default {
                  n224 = Format Into String(format string="%.;:CALC:USER:TRAC8:BDM:X:STAR %g;\n%.;:CALC:USER:TRAC8:BDM:X:STOP %g;", w867, w868) -> (resulting string=w865:string)  [unwired: 2 in, 1 out]
                }
                frame "Span/Center" {
                  n225 = Format Into String(format string="%.;:CALC:USER:TRAC8:BDM:X:CENT %g;\n%.;:CALC:USER:TRAC8:BDM:X:SPAN %g;", w871, w870) -> (resulting string=w869:string)  [unwired: 2 in, 1 out]
                }
              }
              n226 = Select(t=":CALC:USER:TRAC8:BDM:X:STAT ON;", s=w857, f=":CALC:USER:TRAC8:BDM:X:STAT OFF;") -> (s? t:f=w856:string)
              n227 = Concatenate Strings(w856, w860) -> (w861:string)
            }
            frame "Band Marker Y" {
              n228 = case shown="\"Start/Stop\", Default" w881 {
                tunnel: w880 -> [w884 w888]
                tunnel: w879 -> [w885 w887]
                tunnel: [w882 w886] -> w878
                frame "Start/Stop", Default {
                  n229 = Format Into String(format string="%.;:CALC:USER:TRAC8:BDM:Y:STAR %g;\n%.;:CALC:USER:TRAC8:BDM:Y:STOP %g;", w884, w885) -> (resulting string=w882:string)  [unwired: 2 in, 1 out]
                }
                frame "Span/Center" {
                  n230 = Format Into String(format string="%.;:CALC:USER:TRAC8:BDM:Y:CENT %g;\n%.;:CALC:USER:TRAC8:BDM:Y:SPAN %g;", w888, w887) -> (resulting string=w886:string)  [unwired: 2 in, 1 out]
                }
              }
              n231 = Select(t=":CALC:USER:TRAC8:BDM:Y:STAT ON;", s=w874, f=":CALC:USER:TRAC8:BDM:Y:STAT OFF;") -> (s? t:f=w873:string)
              n232 = Concatenate Strings(w873, w878) -> (w877:string)
            }
          }
        }
      }
      n233 = Select(t=":CALC:USER:ALLT:BDM:X:COUP:STAT ON;", s=w559, f=":CALC:USER:ALLT:BDM:X:COUP:STAT OFF;") -> (s? t:f=w558:string)
      n234 = Concatenate Strings(w563, w558) -> (w569:string)
    }
  }
  n235 = VISA Write(VISA resource name="VISA resource name", write buffer=w7, error in (no error)="error in (no error)") -> (VISA resource name out=w9:refnum<visa-resource-name>, error out=w8:errorcluster)  [unwired: 1 out]
  n236 = call "Error Query.vi"("error in (no error)"=w8, "VISA resource name"=w9) -> ("error out"=→"error out":errorcluster, "VISA resource name out"=→"VISA resource name out":refnum<visa-resource-name>)  [unwired: 6 in, 2 out]
